vi "Undo.vi"(8 "error in (no error)":errorcluster, 11 "Canvas in":refnum<class "Canvas.lvclass">) -> (0 "error out":errorcluster, 3 "Canvas out":refnum<class "Canvas.lvclass">)   [LabVIEW 2015, in "Canvas.lvclass"]
uses:
  Canvas.lvclass
  Canvas.lvclass/Canvas.ctl
  Graphic/Graphic.lvclass
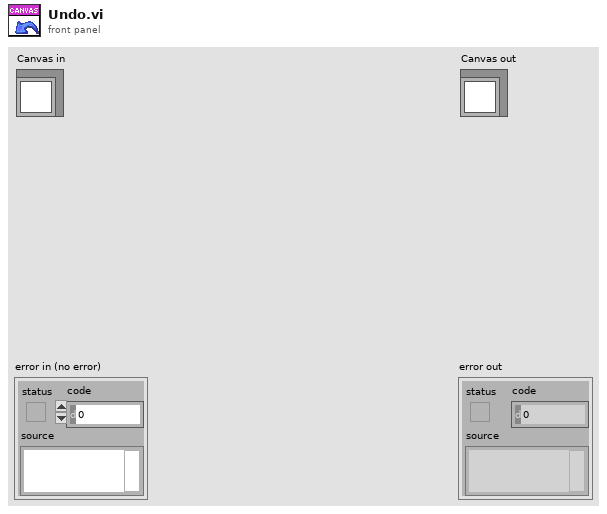
[diagram p1: front panel]
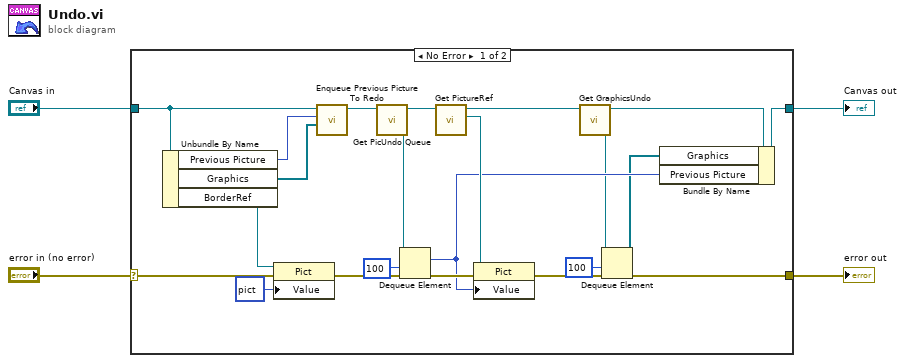
[diagram p0: block diagram]
diagram:
  n1 = case shown="No Error" "error in (no error)" {
    selector: "error in (no error)" -> [w18 w28]
    tunnel: [w7 w28] -> w3
    tunnel: [w20 w27] -> w1
    tunnel: "Canvas in" -> [w16 w27]
    frame No Error {
      n2 = Unbundle By Name(w16) -> ("Previous Picture"=w12:picture, "Graphics"=w11:refnum<class "Graphic.lvclass">[], "BorderRef"=w15:refnum<vi>)
      n3 = property class="Pict"(reference=w15, error in=w18, "Value"=picture data[5B]) -> (error out=w17:errorcluster)  [unwired: 1 out]
      n4 = call "Enqueue Previous Picture To Redo.vi"("Graphic"=w11, "Previous Picture"=w12, "Canvas in"=w16) -> ("Canvas out"=w13:refnum<class "Canvas.lvclass">)  [unwired: 7 in, 1 out]
      n5 = call "Get PicUndo Queue.vi"("Canvas in"=w13) -> ("Undo Queue"=w25:refnum<queue>, "Canvas out"=w26:refnum<class "Canvas.lvclass">)  [unwired: 8 in, 1 out]
      n6 = Dequeue Element(queue=w25, timeout in ms (-1)=100, error in (no error)=w17) -> (element=w19:picture, error out=w21:errorcluster)  [unwired: 2 out]
      n7 = call "Get PictureRef.vi"("Canvas in"=w26) -> ("PictureRef"=w22:refnum<vi>, "Canvas out"=w23:refnum<class "Canvas.lvclass">)  [unwired: 8 in, 1 out]
      n8 = property class="Pict"(reference=w22, error in=w21, "Value"=w19) -> (error out=w8:errorcluster)  [unwired: 1 out]
      n9 = call "Get GraphicsUndo.vi"("Canvas in"=w23) -> ("GraphicsUndo"=w6:refnum<queue>, "Canvas out"=w10:refnum<class "Canvas.lvclass">)  [unwired: 8 in, 1 out]
      n10 = Dequeue Element(queue=w6, timeout in ms (-1)=100, error in (no error)=w8) -> (element=w5:refnum<class "Graphic.lvclass">[], error out=w7:errorcluster)  [unwired: 2 out]
      n11 = Bundle By Name(cluster=w10, "Graphics"=w5, "Previous Picture"=w19) -> (w20:refnum<class "Canvas.lvclass">)
    }
    frame Error {
    }
  }
  "error out" <- w3
  "Canvas out" <- w1
